vi "SSL_get_verify_result.vi"(8 "error in (no error)":errorcluster, 11 "SSL-Lib in":refnum<class "SSL.lvclass">) -> (0 "error out":errorcluster, 2 "verify result":T1, 3 "SSL-Lib out":refnum<class "SSL.lvclass">)   [LabVIEW 2013, in "SSL_Lib.lvlib" / "SSL.lvclass"]
uses:
  SSL.lvclass
  X509_Verify_Result.ctl
  SSL-Lib/SSL-Lib.lvclass/SSL-Lib.ctl
  SSL.lvclass/SSL.ctl
  SSL-Lib/Read SSL Library Path.vi
  Read Handle.vi
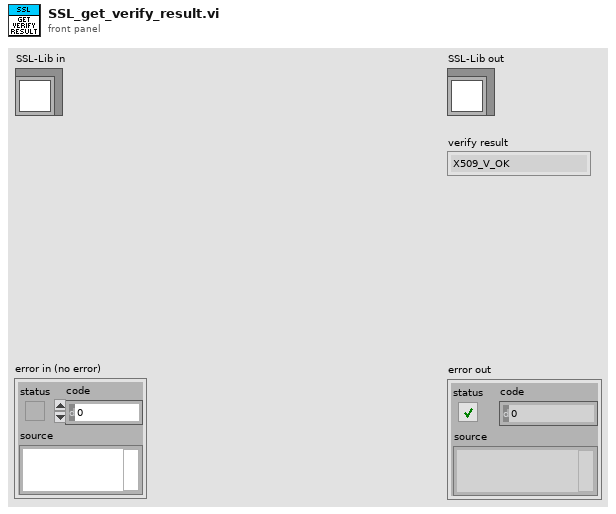
[diagram p1: front panel]
types:
  T1 = typedef "SSL_Lib.lvlib/SSL.lvclass/X509_Verify_Result.ctl" = enum16{"X509_V_OK", "X509_V_ERR_UNSPECIFIED", "X509_V_ERR_UNABLE_TO_GET_ISSUER_CERT", "X509_V_ERR_UNABLE_TO_GET_CRL", "X509_V_ERR_UNABLE_TO_DECRYPT_CERT_SIGNATURE", "X509_V_ERR_UNABLE_TO_DECRYPT_CRL_SIGNATURE", "X509_V_ERR_UNABLE_TO_DECODE_ISSUER_PUBLIC_KEY", "X509_V_ERR_CERT_SIGNATURE_FAILURE", "X509_V_ERR_CRL_SIGNATURE_FAILURE", "X509_V_ERR_CERT_NOT_YET_VALID", "X509_V_ERR_CERT_HAS_EXPIRED", "X509_V_ERR_CRL_NOT_YET_VALID", "X509_V_ERR_CRL_HAS_EXPIRED", "X509_V_ERR_ERROR_IN_CERT_NOT_BEFORE_FIELD", "X509_V_ERR_ERROR_IN_CERT_NOT_AFTER_FIELD", "X509_V_ERR_ERROR_IN_CRL_LAST_UPDATE_FIELD", "X509_V_ERR_ERROR_IN_CRL_NEXT_UPDATE_FIELD", "X509_V_ERR_OUT_OF_MEM", "X509_V_ERR_DEPTH_ZERO_SELF_SIGNED_CERT", "X509_V_ERR_SELF_SIGNED_CERT_IN_CHAIN", "X509_V_ERR_UNABLE_TO_GET_ISSUER_CERT_LOCALLY", "X509_V_ERR_UNABLE_TO_VERIFY_LEAF_SIGNATURE", "X509_V_ERR_CERT_CHAIN_TOO_LONG", "X509_V_ERR_CERT_REVOKED", "X509_V_ERR_INVALID_CA", "X509_V_ERR_PATH_LENGTH_EXCEEDED", "X509_V_ERR_INVALID_PURPOSE", "X509_V_ERR_CERT_UNTRUSTED", "X509_V_ERR_CERT_REJECTED", "X509_V_ERR_SUBJECT_ISSUER_MISMATCH", "X509_V_ERR_AKID_SKID_MISMATCH", "X509_V_ERR_AKID_ISSUER_SERIAL_MISMATCH", "X509_V_ERR_KEYUSAGE_NO_CERTSIGN", "X509_V_ERR_UNABLE_TO_GET_CRL_ISSUER", "X509_V_ERR_UNHANDLED_CRITICAL_EXTENSION", "X509_V_ERR_KEYUSAGE_NO_CRL_SIGN", "X509_V_ERR_UNHANDLED_CRITICAL_CRL_EXTENSION", "X509_V_ERR_INVALID_NON_CA", "X509_V_ERR_PROXY_PATH_LENGTH_EXCEEDED", "X509_V_ERR_KEYUSAGE_NO_DIGITAL_SIGNATURE", "X509_V_ERR_PROXY_CERTIFICATES_NOT_ALLOWED", "X509_V_ERR_INVALID_EXTENSION", "X509_V_ERR_INVALID_POLICY_EXTENSION", "X509_V_ERR_NO_EXPLICIT_POLICY", "X509_V_ERR_DIFFERENT_CRL_SCOPE", "X509_V_ERR_UNSUPPORTED_EXTENSION_FEATURE", "X509_V_ERR_UNNESTED_RESOURCE", "X509_V_ERR_PERMITTED_VIOLATION", "X509_V_ERR_EXCLUDED_VIOLATION", "X509_V_ERR_SUBTREE_MINMAX", "X509_V_ERR_APPLICATION_VERIFICATION", "X509_V_ERR_UNSUPPORTED_CONSTRAINT_TYPE", "X509_V_ERR_UNSUPPORTED_CONSTRAINT_SYNTAX", "X509_V_ERR_UNSUPPORTED_NAME_SYNTAX", "X509_V_ERR_CRL_PATH_VALIDATION_ERROR", "N/A", "X509_V_ERR_SUITE_B_INVALID_VERSION", "X509_V_ERR_SUITE_B_INVALID_ALGORITHM", "X509_V_ERR_SUITE_B_INVALID_CURVE", "X509_V_ERR_SUITE_B_INVALID_SIGNATURE_ALGORITHM", "X509_V_ERR_SUITE_B_LOS_NOT_ALLOWED", "X509_V_ERR_SUITE_B_CANNOT_SIGN_P_384_WITH_P_256", "X509_V_ERR_HOSTNAME_MISMATCH", "X509_V_ERR_EMAIL_MISMATCH", "X509_V_ERR_IP_ADDRESS_MISMATCH", "X509_V_ERR_INVALID_CALL", "X509_V_ERR_STORE_LOOKUP", "X509_V_ERR_PROXY_SUBJECT_NAME_VIOLATION"}
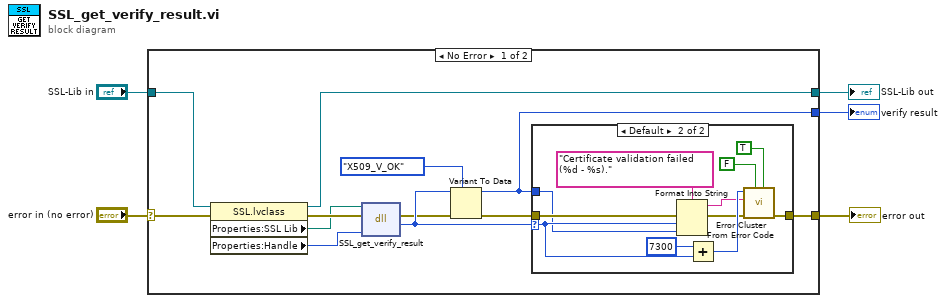
[diagram p0: block diagram]
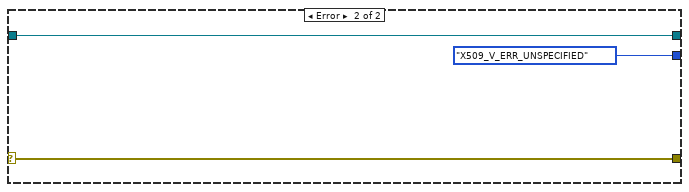
[diagram p3: hidden frame]
diagram:
  n1 = case shown="No Error" "error in (no error)" {
    selector: "error in (no error)" -> [w17 w31]
    tunnel: [w12 w32] -> w3
    tunnel: "SSL-Lib in" -> [w13 w32]
    tunnel: [w10 w31] -> w2
    tunnel: [w8 X509_Verify_Result."X509_V_ERR_UNSPECIFIED"] -> w1
    frame No Error {
      n2 = property class="SSL.lvclass"(reference=w13, error in=w17) -> (reference out=w12:refnum<class "SSL.lvclass">, error out=w16:errorcluster, "Properties:SSL Lib"=w15:path, "Properties:Handle"=w14:u64)
      n3 = dll-call lib="C:/Program Files (x86)/National Instruments/Shared/nissl/NIssleay32.dll" fn="SSL_get_verify_result"(path in=w15, error in=w16, "SSL"=w14) -> (error out=w7:errorcluster, "return type"=w9:i32)  [unwired: 2 in, 1 out]
      n4 = Variant To Data(error in=w7, type=X509_Verify_Result."X509_V_OK", Variant=w9) -> (data=w8:T1, error out=w6:errorcluster)
      n5 = case shown="Default" w9 {
        selector: w9 -> [_ w21]
        tunnel: w8 -> [_ w20]
        tunnel: w6 -> [w18 w29]
        tunnel: [w18 w28] -> w10
        frame 0 {
        }
        frame Default {
          n6 = Format Into String(format string="Certificate validation failed (%d - %s).", error in=w29, w21, w20) -> (resulting string=w25:string, error out=w24:errorcluster)  [unwired: 1 in]
          n7 = Add(x=7300, y=w21) -> (x+y=w27:i32)
          n8 = call <vilib>:"Error Cluster From Error Code.vi"("is warning? (False)"=TRUE, "show call chain? (False)"=FALSE, "error in (no error)"=w24, "error message (\"\")"=w25, "error code (0)"=w27) -> ("error out"=w28:errorcluster)  [unwired: 4 in]
        }
      }
    }
    frame Error {
    }
  }
  "SSL-Lib out" <- w3
  "error out" <- w2
  "verify result" <- w1
